vi "generate table.vi"(7 "table":T1, 8 "error in":errorcluster, 10 "engine configuration":refnum<class "engine configuration.lvclass">, 11 "tag bus configurable plugin module configuration":refnum<class "UI Reference configuration.lvclass">) -> (0 "error out":errorcluster)   [LabVIEW 2013, in "UI Reference editor node.lvclass"]
uses:
  UI Reference editor node.lvclass
  table reference.ctl
  module/configuration/UI Reference configuration.lvclass
  <vilib>/NI/Module Execution Interface/Engine Configuration/engine configuration.lvclass
  <vilib>/NI/Tag Bus Module Framework/root configuration/TBM configuration.lvclass/TBM configuration.ctl
  table line.ctl
  <vilib>/NI/Tag Bus Module Framework/channel/TBM channel.lvclass
  <vilib>/NI/Tag Bus/tag/tag descriptor.lvclass/tag descriptor.ctl
  <vilib>/NI/Tag Bus/tag/read tag name.vi
  <vilib>/NI/Tag Bus Module Framework/root configuration/Read instance name.vi
  <vilib>/NI/Tag Bus Module Framework/root configuration/create GUID.vi
  <vilib>/NI/Tag Bus/tag/tag descriptor.lvclass
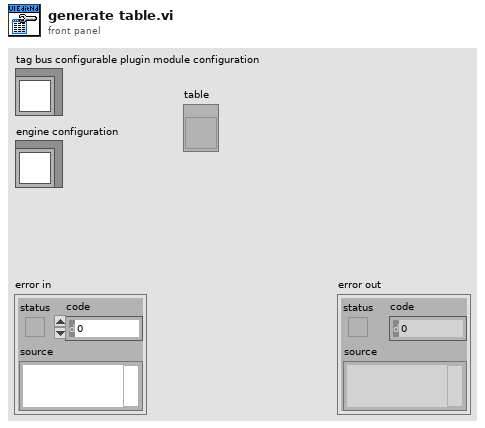
[diagram p1: front panel]
types:
  T1 = typedef "UI Reference editor node.lvclass/table reference.ctl" = refnum<vi>
  T2 = typedef "UI Reference editor node.lvclass/table line.ctl" = cluster{"channel":refnum<class "TBM channel.lvclass">, "tag name":string}
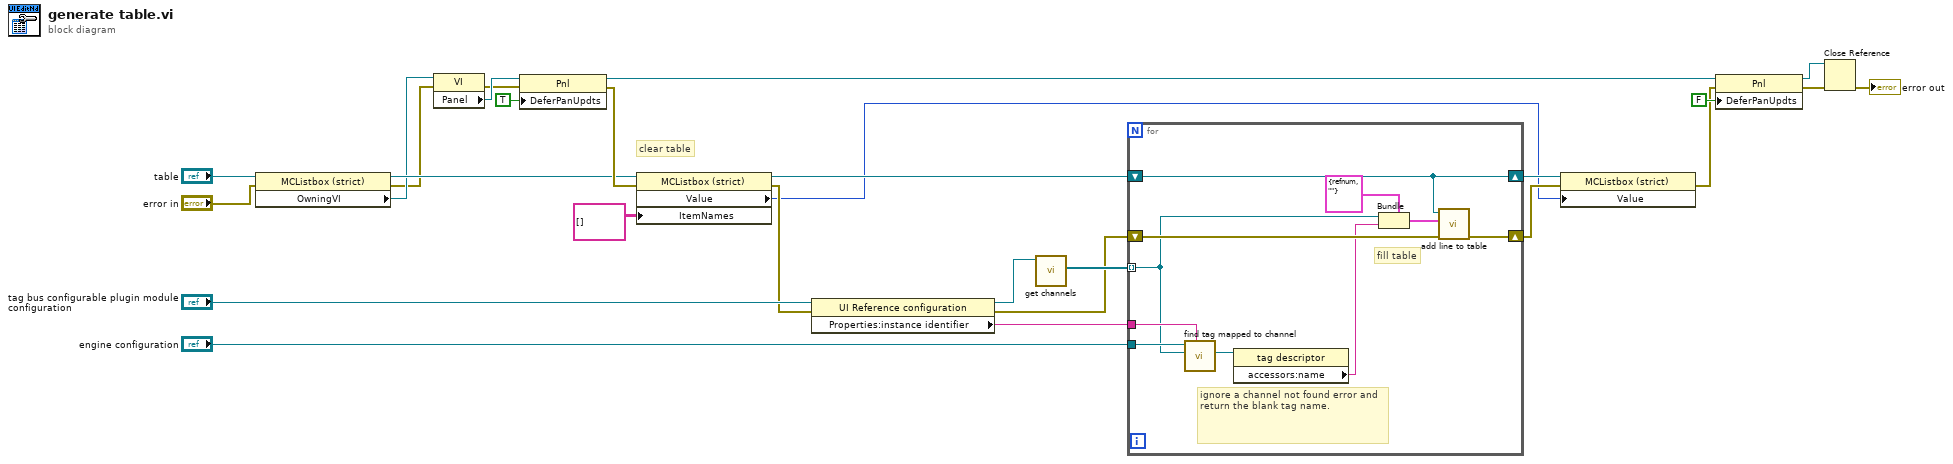
[diagram p0: block diagram]
diagram:
  # "clear table"
  n1 = property class="MCListbox (strict)"(reference="table", error in="error in") -> (reference out=w6:T1, error out=w3:errorcluster, "OwningVI"=w4:refnum<vi>)
  n2 = property class="VI"(reference=w4, error in=w3) -> (error out=w12:errorcluster, "Panel"=w13:refnum<vi>)  [unwired: 1 out]
  n3 = property class="Pnl"(reference=w13, error in=w12, "DeferPanUpdts"=TRUE ("Defer Panel Updates")) -> (reference out=w9:refnum<vi>, error out=w11:errorcluster)
  n4 = property class="MCListbox (strict)"(reference=w6, error in=w11, "ItemNames"=string[][] [] ("Item Names")) -> (reference out=w25:T1, error out=w20:errorcluster, "Value"=w15:i32)
  n5 = property class="UI Reference configuration"(reference="tag bus configurable plugin module configuration", error in=w20) -> (reference out=w22:refnum<class "UI Reference configuration.lvclass">, error out=w19:errorcluster, "Properties:instance identifier"=w21:string)
  n6 = call-dynamic "get channels.vi"("UI Reference configuration in"=w22) -> ("channels"=w26:refnum<class "TBM channel.lvclass">[])  [unwired: 9 in, 1 out]
  n7 = for {
    shift-right: [w37] -> w16
    shift-left: w19 -> [w34]
    tunnel: w26 -> [w31] mode=indexing
    tunnel: "engine configuration" -> [w33]
    tunnel: w21 -> [w32]
    shift-right: [w28] -> w17
    shift-left: w25 -> [w28]
    # "ignore a channel not found error and return the blank tag name."
    # "fill table"
    n8 = call <vilib>:"find tag mapped to channel.vi"("owner"=w32, "channel"=w31, "engine configuration in"=w33) -> ("tag"=w30:refnum<class "tag descriptor.lvclass">)  [unwired: 6 in, 2 out]
    n9 = property class="tag descriptor"(reference=w30) -> ("accessors:name"=w29:string)  [unwired: 1 in, 2 out]
    n10 = Bundle(cluster=T2 {"channel"=refnum, "tag name"=""} ("line"), "channel"=w31, "tag name"=w29) -> (w35:T2)
    n11 = call "add line to table.vi"("error in"=w34, "line"=w35, "operations table"=w28) -> ("error out"=w37:errorcluster)  [unwired: 8 in]
  }
  n12 = property class="MCListbox (strict)"(reference=w17, error in=w16, "Value"=w15) -> (error out=w8:errorcluster)  [unwired: 1 out]
  n13 = property class="Pnl"(reference=w9, error in=w8, "DeferPanUpdts"=FALSE ("Defer Panel Updates")) -> (reference out=w1:refnum<vi>, error out=w7:errorcluster)
  n14 = Close Reference(reference=w1, error in (no error)=w7) -> (error out=→"error out":errorcluster)
